vi "JX_MoveBySteps.vi"(6 "Direction":bool, 7 "Channel":u8, 8 "error in (no error)":errorcluster, 9 "Steps":u16, 11 "MB Serial Master:MB_Master":refnum<class "MB_Master.lvclass">) -> (0 "error out":errorcluster, 3 "MB Serial Master:MB_Master":refnum<class "MB_Master.lvclass">)   [LabVIEW 2023, in "TranslationStage Library.lvlib" / "Jiaxin_Stepper_Controller.lvlib"]
uses:
  Jiaxin_Stepper_Controller.lvlib
  <vilib>/Plasmionique/MB Master/MB_Master/MB_Master.lvclass
  <vilib>/Plasmionique/MB Master/MB Master.lvlib
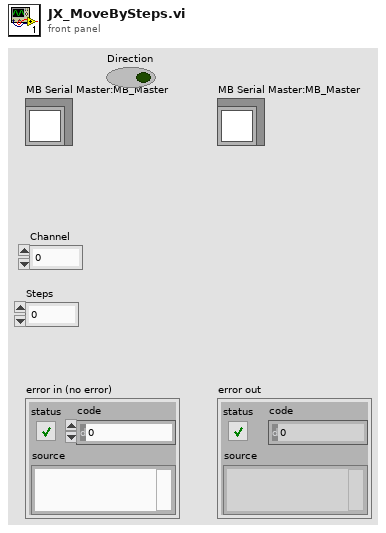
[diagram p1: front panel]
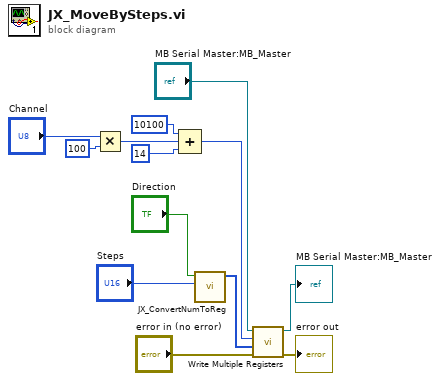
[diagram p0: block diagram]
diagram:
  n1 = Multiply(x="Channel", y=u16 100) -> (x*y=w8:u16)
  n2 = Compound Arithmetic op=ADD(u16 10100 ("value"), w8, u8 14 ("value")) -> (w3:u16)
  n3 = call "JX_ConvertNumToReg.vi"("Steps"="Steps", "Direction"="Direction") -> ("Array"=w10:u16[])  [unwired: 9 in]
  n4 = call <vilib>:"Write Multiple Registers.vi"("error in (no error)"="error in (no error)", "values"=w10, "starting address"=w3, "MB session in"="MB Serial Master:MB_Master") -> ("error out"=→"error out":errorcluster, "MB session out"=→"MB Serial Master:MB_Master":refnum<class "MB_Master.lvclass">)  [unwired: 6 in]
